vi "Tatrocki_prac9.vi"() -> ()   [LabVIEW 2023]
uses:
  <vilib>/Platform/TimedLoop/XDataNode/timing_clust.ctl
  <vilib>/Platform/TimedLoop/XDataNode/nitl_modes.ctl
  <vilib>/Platform/TimedLoop/XDataNode/wakeup.ctl
  <vilib>/Platform/TimedLoop/scheduler/LVUserAPI/_suppVIs/Create_1kHz_TSource.vi
  <vilib>/platform/TimedLoop/XDataNode/XDataNode.xnode
  <vilib>/Platform/TimedLoop/XDataNode/XDNodeRunTimeDep.lvlib
panel:
  in  "Synchronizacja":bool
  out "L2 Stop":u32
  out "?":bool
  out "Numer Petli 2":i64
  out "L2 End":i64
  out "L1 Stop":dbl
  out "Czas poczatkowy":u32
  out "?":bool
  out "Numer petli 1":dbl
  out "L1 End":i64
  in  "Okres (s)":dbl=0.5 min=0.5 max=20.0 step=0.5
  out "S0 End":i64
  out "SO Start":i64
  out "Error 2":errorcluster
  out "Error 1":errorcluster
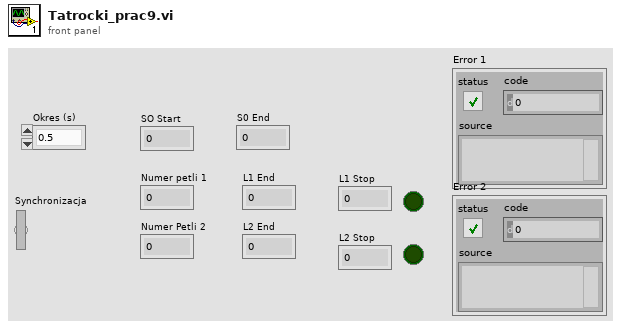
[diagram p1: front panel]
types:
  T1 = typedef "XDNodeRunTimeDep.lvlib/timing_clust.ctl" = cluster{"Expected End [f-1]":u64, "Actual End [f-1]":u64, "Finished Late? [f-1]":bool, "Expected End [i-1]":u64, "Actual End [i-1]":u64, "Finished Late? [i-1]":bool, "Expected Start [i]":u64, "Actual Start [i]":u64, "Expected Start [f]":u64, "Actual Start [f]":u64, "Source Name":string, "Structure Name":string, "Period":i64, "Deadline":i64, "Offset":i64, "Start":i64, "Priority":i32, "Timeout":i32, "Mode":T2, "Wakeup Reason":T3, "Error":errorcluster, "Source Type":string, "Secondary Source Type":string, "Global End Time":u64, "Global Start Time":u64, "Frame Duration":u64, "Iteration Duration":u64, "Assigned CPU":i32, "I/O Scan Engine Mode":u32}
  T2 = typedef "XDNodeRunTimeDep.lvlib/nitl_modes.ctl" = enum32{"No Change", "Process missed periods, maintain original phase", "Discard missed periods, maintain original phase", "Process missed periods, ignore original phase", "Discard missed periods, ignore original phase"}
  T3 = typedef "XDNodeRunTimeDep.lvlib/wakeup.ctl" = enum32{"Normal", "Aborted", "Asynchronous wakeup", "Timing source error", "Timed loop error", "Timeout"}
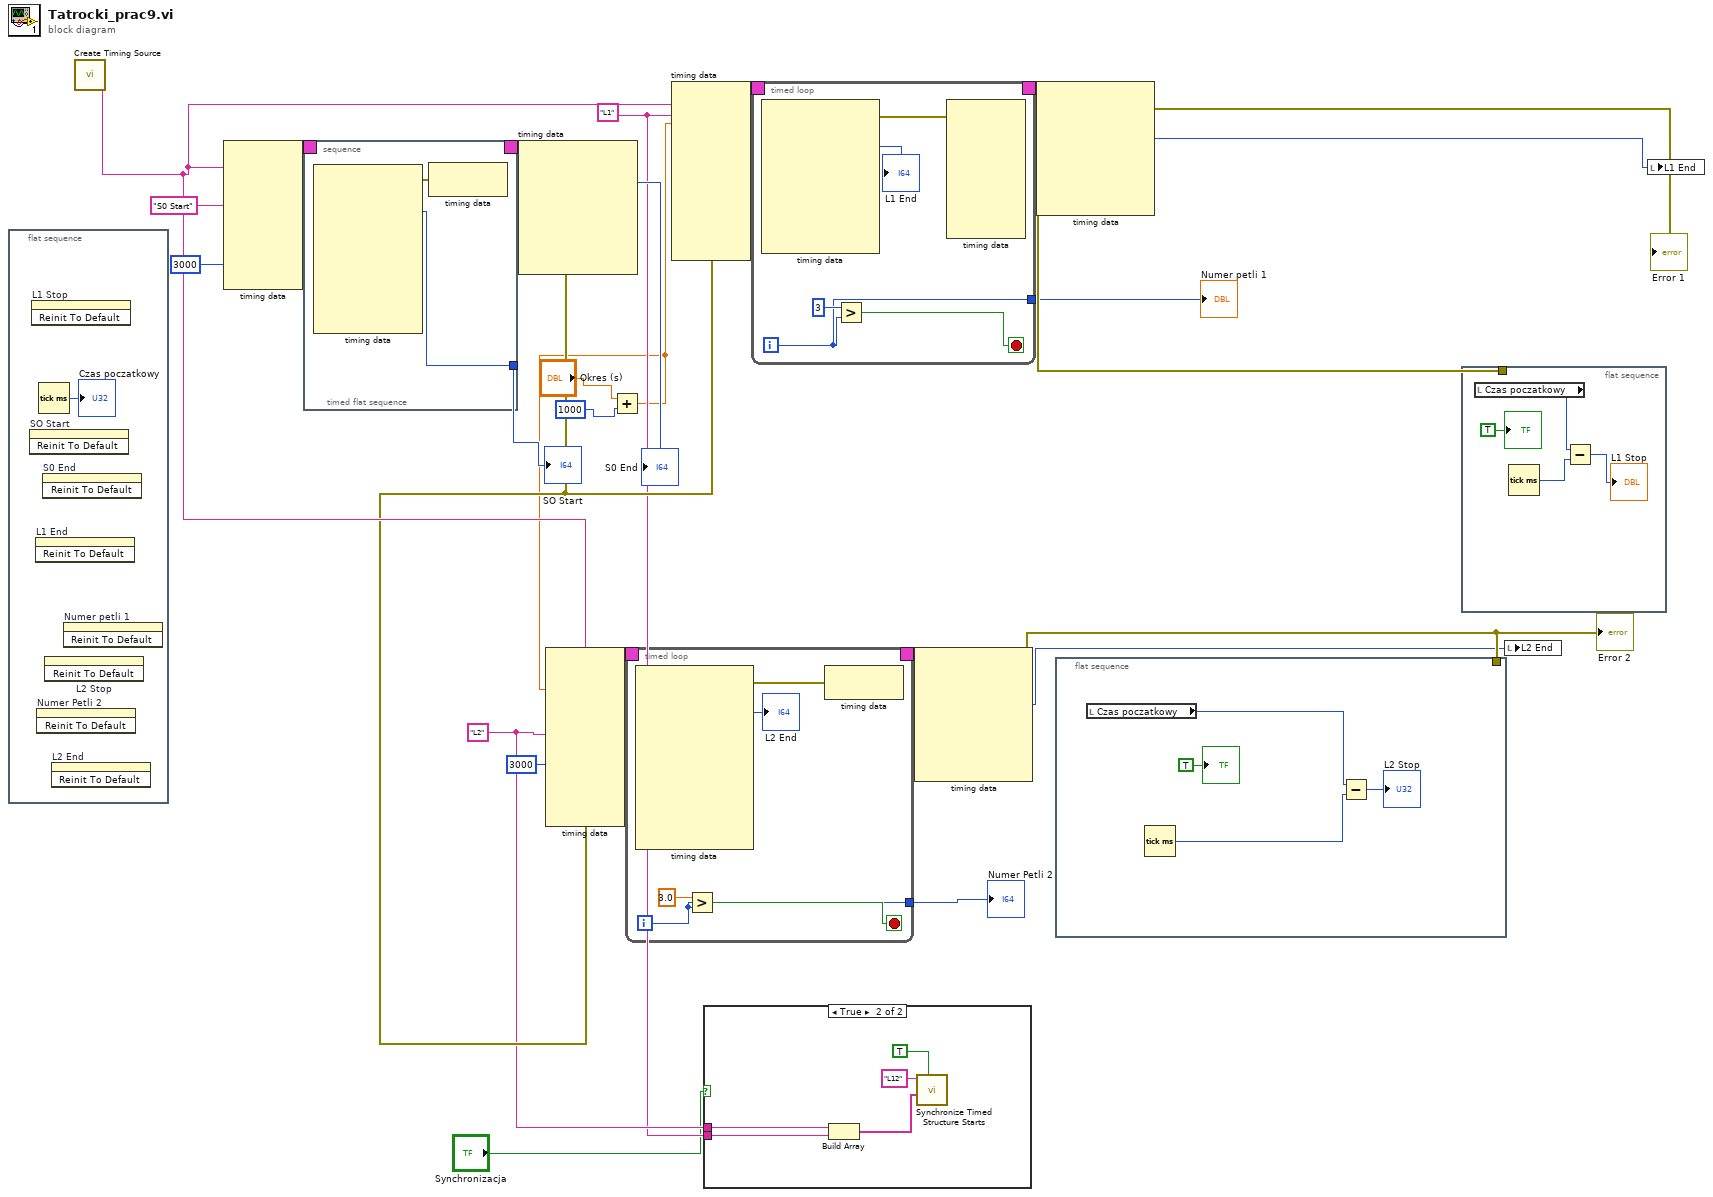
[diagram p0: block diagram]
diagram:
  w6 = "L2" ("Structure Name")
  w5 = "L1" ("Structure Name")
  n1 = flat-sequence {
    frame #0 {
      n2 = invoke on="SO Start" class="DigNum (strict)" method="Reinit To Default"() -> ()  [unwired: 3 in, 3 out]
      n3 = invoke on="L1 Stop" class="DigNum (strict)" method="Reinit To Default"() -> ()  [unwired: 3 in, 3 out]
      n4 = invoke on="L1 End" class="DigNum (strict)" method="Reinit To Default"() -> ()  [unwired: 3 in, 3 out]
      n5 = invoke on="Numer Petli 2" class="DigNum (strict)" method="Reinit To Default"() -> ()  [unwired: 3 in, 3 out]
      n6 = Tick Count (ms)() -> (millisecond timer value=→"Czas poczatkowy":u32)
      n7 = invoke on="S0 End" class="DigNum (strict)" method="Reinit To Default"() -> ()  [unwired: 3 in, 3 out]
      n8 = invoke on="L2 Stop" class="DigNum (strict)" method="Reinit To Default"() -> ()  [unwired: 3 in, 3 out]
      n9 = invoke on="L2 End" class="DigNum (strict)" method="Reinit To Default"() -> ()  [unwired: 3 in, 3 out]
      n10 = invoke on="Numer petli 1" class="DigNum (strict)" method="Reinit To Default"() -> ()  [unwired: 3 in, 3 out]
    }
  }
  n11 = call-poly <vilib>:"Create Timing Source.vi"() -> ("name (out)"=w10:string)  [unwired: 10 in, 1 out]
  n12 = node-c288(w10, "S0 Start" ("Structure Name"), u32 3000 ("milliseconds to wait")) -> (w21:T1)  [unwired: 5 in]
  n13 = timed-sequence {
    timing: w21 -> [_]
    timing-out: [_] -> w20
    tunnel: [w27] -> w15
    n14 = timed-flat-sequence {
      tunnel: [w28] -> w27
      n15 = node-c288() -> (w29:errorcluster, w28:i64)  [unwired: 1 in, 8 out]
      n16 = node-c288(w29) -> ()  [unwired: 1 out]
    }
  }
  "SO Start" <- w15
  n17 = node-c288(w20) -> (w8:errorcluster, →"S0 End":i64)  [unwired: 5 out]
  n18 = Add(x="Okres (s)", y=1000) -> (x+y=w3:dbl)
  n19 = node-c288(w10, w3, w6, i64 3000 ("Offset"), w8) -> (w23:T1)  [unwired: 5 in]
  n20 = timed-loop {
    timing: w23 -> [_]
    timing-out: [_] -> w22
    tunnel: [w36] -> w2
    i -> [w36]
    stop <- w37 stop-if-true
    n21 = node-c288() -> (w40:errorcluster, →"L2 End":i64)  [unwired: 1 in, 9 out]
    n22 = Greater?(x=3.0, y=w36) -> (0:w37:bool)
    n23 = node-c288(w40) -> ()  [unwired: 1 out]
  }
  "Numer Petli 2" <- w2
  n24 = node-c288(w10, w3, w5, w8) -> (w25:T1)  [unwired: 6 in]
  n25 = case shown="True" "Synchronizacja" {
    tunnel: w6 -> [_ w48]
    tunnel: w5 -> [_ w47]
    frame False {
    }
    frame True {
      n26 = Build Array(w48, w47) -> (w49:string[])
      n27 = call <vilib>:"Synchronize Timed Structure Starts.vi"("replace (T)"=TRUE, "timed structure names"=w49, "synchronization group name"="L12") -> ()  [unwired: 7 in, 2 out]
    }
  }
  n28 = timed-loop {
    timing: w25 -> [_]
    timing-out: [_] -> w24
    tunnel: [w52] -> w1
    i -> [w52]
    stop <- w53 stop-if-true
    n29 = node-c288() -> (w56:errorcluster, →"L1 End":i64)  [unwired: 1 in, 7 out]
    n30 = Greater?(x=3, y=w52) -> (0:w53:bool)
    n31 = node-c288(w56) -> ()  [unwired: 7 in, 1 out]
  }
  "Numer petli 1" <- w1
  n32 = node-c288(w22) -> (w18:errorcluster, w7:i64)  [unwired: 5 out]
  "Error 2" <- w18
  n33 = node-c288(w24) -> (w19:errorcluster, w11:i64)  [unwired: 5 out]
  "Error 1" <- w19
  n34 = flat-sequence {
    tunnel: w18 -> [_]
    frame #0 {
      n35 = local read "Czas poczatkowy"() -> (w65:u32)
      n36 = Tick Count (ms)() -> (millisecond timer value=w64:u32)
      n37 = Subtract(x=w65, y=w64) -> (x-y=→"L2 Stop":u32)
      "?" <- TRUE ("Boolean")
    }
  }
  n38 = flat-sequence {
    tunnel: w19 -> [_]
    frame #0 {
      n39 = local read "Czas poczatkowy"() -> (w69:u32)
      n40 = Tick Count (ms)() -> (millisecond timer value=w68:u32)
      n41 = Subtract(x=w69, y=w68) -> (x-y=→"L1 Stop":u32)
      "?" <- TRUE ("Boolean")
    }
  }
  n42 = local write "L2 End"(w7) -> ()
  n43 = local write "L1 End"(w11) -> ()
